vi "RoundToFixedDPs.vi"(9 "Power of ten":i32, 11 "Number to round":dbl=1234.56789 format="%_9f") -> (1 "Decimal place":dbl=1.0 format="%#_9f", 3 "Rounded number":dbl=1235.0 format="%_9f")   [LabVIEW 2021]
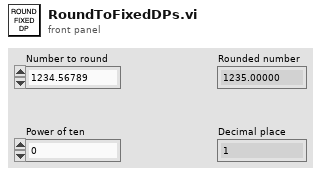
[diagram p1: front panel]
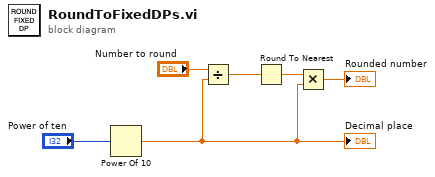
[diagram p0: block diagram]
diagram:
  n1 = Power Of 10(x="Power of ten") -> (10^x=w6:dbl)
  "Decimal place" <- w6
  n2 = Divide(x="Number to round", y=w6) -> (x/y=w3:dbl)
  n3 = Round To Nearest(number=w3) -> (nearest integer value=w4:dbl)
  n4 = Multiply(x=w4, y=w6) -> (x*y=→"Rounded number":dbl)
